vi "WORD report.vi"(7 "Action":T1=enum."Close report", 8 "error in":errorcluster, 10 "Data in":string) -> (0 "error out":errorcluster, 2 "Data out":variant)   [LabVIEW 2015, in "Report.lvlib"]
uses:
  Report.lvlib
  TypeDefs/Report state.ctl
  <vilib>/Utility/NIReport.llb/NI_report.lvclass
  <vilib>/Utility/NIReport.llb/Append Report Text (str wrap).vi
  <vilib>/Utility/NIReport.llb/NI_ReportGenerationCore.lvlib
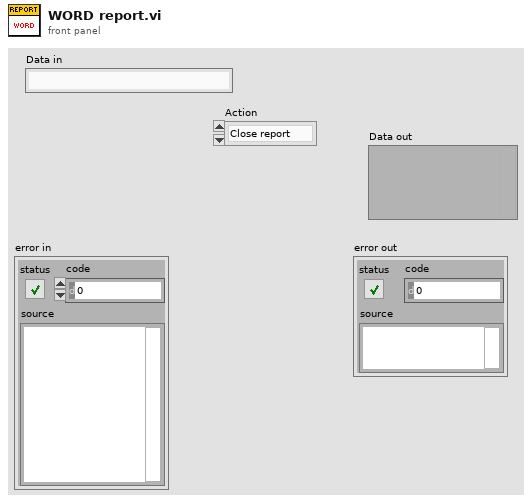
[diagram p1: front panel]
types:
  T1 = typedef "Report.lvlib/Report state.ctl" = enum16{"Create report", "Save data", "Save report", "Available printers", "Print report", "Close report"}
  T2 = enum16{"maximized", "minimized", "normal", "no change"}
  T3 = enum16{"Standard Report", "HTML", "Word", "Excel"}
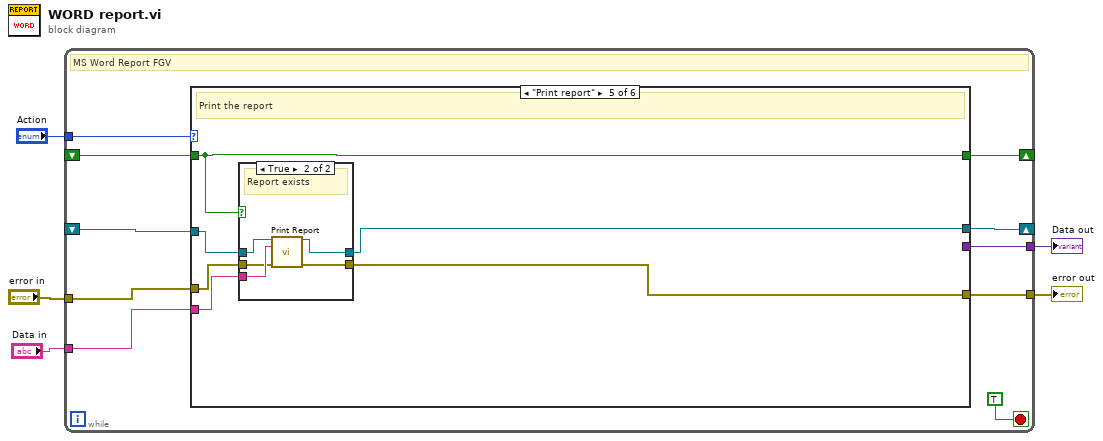
[diagram p0: block diagram]
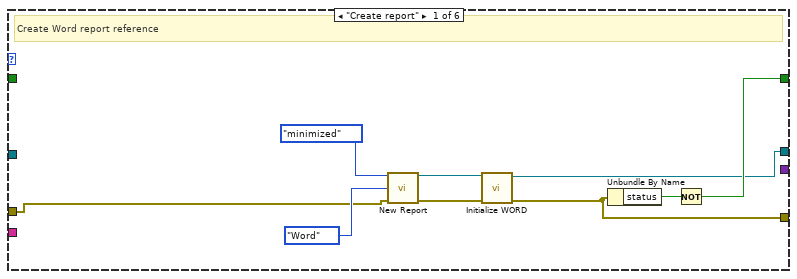
[diagram p2: hidden frame]
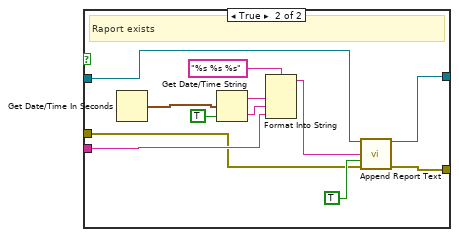
[diagram p4: hidden frame]
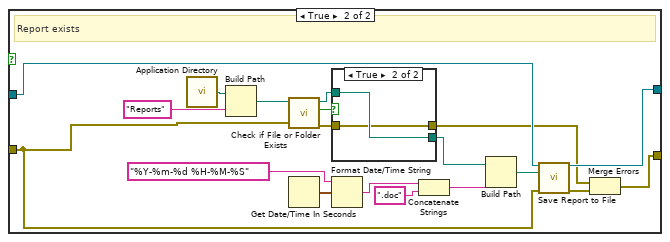
[diagram p6: hidden frame]
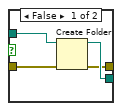
[diagram p7: hidden frame]
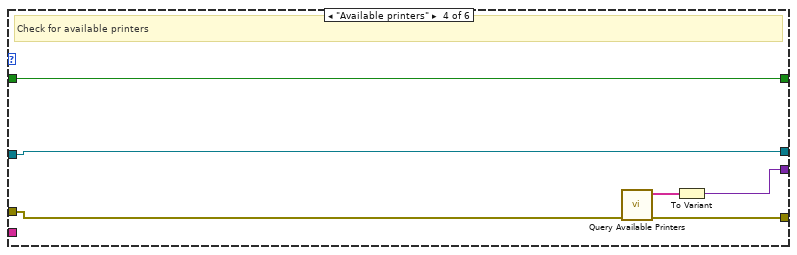
[diagram p8: hidden frame]
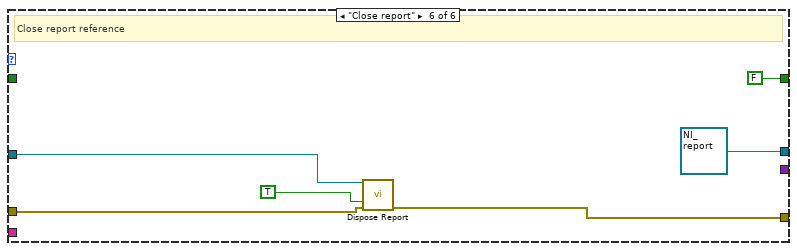
[diagram p10: hidden frame]
diagram:
  n1 = while {
    tunnel: "Action" -> [w13]
    tunnel: "Data in" -> [w14]
    tunnel: "error in" -> [w12]
    tunnel: [w11] -> w3
    tunnel: [w10] -> w1
    shift-right: [w8] -> _
    shift-left: _ -> [w9]
    shift-right: [w7] -> _
    shift-left: _ -> [w6]
    stop <- TRUE stop-if-true
    # "MS Word Report FGV"
    n2 = case shown="\"Print report\"" w13 {
      tunnel: w14 -> [_ w30 _ _ w88 _]
      tunnel: w12 -> [w20 w27 w47 w80 w85 w96]
      tunnel: [_ _ _ w81 _ _] -> w11
      tunnel: [w19 w29 w49 w79 w87 w101] -> w10
      tunnel: w9 -> [_ w28 w48 w78 w86 _]
      tunnel: [w17 w28 w48 w78 w86 FALSE] -> w8
      tunnel: [w16 w25 w45 w77 w83 refnum<class "NI_report.lvclass"> refnum ("report ID")] -> w7
      tunnel: w6 -> [_ w26 w46 w77 w84 w98]
      frame "Create report" {
        # "Create Word report reference"
        n3 = call <vilib>:"New Report.vi"("window state (normal)"=T2."minimized", "report type"=T3."Word", "error in (no error)"=w20) -> ("report out"=w22:refnum<class "NI_report.lvclass">, "error out"=w21:errorcluster)  [unwired: 11 in]
        n4 = call "Initialize WORD.vi"("error in (no error)"=w21, "NI_report in"=w22) -> ("error out"=w19:errorcluster, "NI_report out"=w16:refnum<class "NI_report.lvclass">)  [unwired: 8 in]
        n5 = Unbundle By Name(w19) -> ("status"=w18:bool)
        n6 = Not(x=w18) -> (.not. x?=w17:bool)
      }
      frame "Save data" {
        # "Save date, time and input message (status) in new line"
        n7 = case shown="False" w28 {
          tunnel: w30 -> [_ w37]
          tunnel: [w32 w36] -> w29
          tunnel: w27 -> [w32 w33]
          tunnel: w26 -> [w31 w35]
          tunnel: [w31 w34] -> w25
          frame False {
            # "Report not created"
          }
          frame True {
            # "Raport exists"
            n8 = Get Date/Time In Seconds() -> (seconds since 1Jan1904=w43:timestamp)
            n9 = Get Date/Time String(seconds (now)=w43, want seconds? (F)=TRUE) -> (date string=w41:string, time string=w40:string)  [unwired: 1 in]
            n10 = Format Into String(format string="%s %s %s", w41, w40, w37) -> (resulting string=w38:string)  [unwired: 2 in, 1 out]
            n11 = call-poly <vilib>:"Append Report Text.vi"("report in"=w35, "text"=w38, "append on new line? (F)"=TRUE ("append on new line?"), "error in (no error)"=w33) -> ("report out"=w34:refnum<class "NI_report.lvclass">, "error out"=w36:errorcluster)  [unwired: 8 in, 2 out]
          }
        }
      }
      frame "Save report" {
        # "Save report file on HDD"
        n12 = case shown="False" w48 {
          tunnel: [w51 w52] -> w49
          tunnel: w47 -> [w51 w56]
          tunnel: w46 -> [w50 w58]
          tunnel: [w50 w57] -> w45
          frame False {
            # "Report not created"
          }
          frame True {
            # "Report exists"
            n13 = call <vilib>:"Application Directory.vi"() -> ("Application Directory"=w64:path)
            n14 = Build Path(base path=w64, name or relative path="Reports") -> (appended path=w62:path)
            n15 = call <vilib>:"Check if File or Folder Exists.vi"("error in (no error)"=w56, "path"=w62) -> ("error out"=w55:errorcluster, "file or folder exists?"=w61:bool, "dup path"=w60:path)  [unwired: 7 in]
            n16 = Get Date/Time In Seconds() -> (seconds since 1Jan1904=w69:timestamp)
            n17 = case shown="True" w61 {
              tunnel: w60 -> [w74 w76]
              tunnel: [w73 w76] -> w59
              tunnel: w55 -> [w72 w75]
              tunnel: [w71 w75] -> w54
              frame False {
                n18 = Create Folder(path (use dialog)=w74, error in=w72) -> (created path=w73:path, error out=w71:errorcluster)  [unwired: 1 in, 1 out]
              }
              frame True {
              }
            }
            n19 = Format Date/Time String(time format string (%c)="%Y-%m-%d %H-%M-%S", seconds (now)=w69) -> (date/time string=w67:string)  [unwired: 1 in]
            n20 = Concatenate Strings(w67, ".doc" ("string")) -> (w65:string)
            n21 = Build Path(base path=w59, name or relative path=w65) -> (appended path=w70:path)
            n22 = call-dynamic "Save Report to File.vi"("report in"=w58, "report file path"=w70, "error in (no error)"=w56) -> ("report out"=w57:refnum<class "NI_report.lvclass">, "error out"=w53:errorcluster)  [unwired: 11 in]
            n23 = Merge Errors(w54, w53) -> (w52:errorcluster)
          }
        }
      }
      frame "Available printers" {
        # "Check for available printers"
        n24 = call <vilib>:"Query Available Printers.vi"("error in (no error)"=w80) -> ("error out"=w79:errorcluster, "system configured printers"=w82:string[])  [unwired: 8 in, 1 out]
        n25 = To Variant(anything=w82) -> (Variant=w81:variant)
      }
      frame "Print report" {
        # "Print the report"
        n26 = case shown="True" w86 {
          tunnel: w88 -> [_ w95]
          tunnel: [w90 w94] -> w87
          tunnel: w85 -> [w90 w91]
          tunnel: w84 -> [w89 w93]
          tunnel: [w89 w92] -> w83
          frame False {
            # "Report not created"
          }
          frame True {
            # "Report exists"
            n27 = call-dynamic "Print Report.vi"("report in"=w93, "printer name (default)"=w95, "error in (no error)"=w91) -> ("report out"=w92:refnum<class "NI_report.lvclass">, "error out"=w94:errorcluster)  [unwired: 11 in]
          }
        }
      }
      frame "Close report" {
        # "Close report reference"
        n28 = call-dynamic "Dispose Report.vi"("report in"=w98, "save changes? (F)"=TRUE, "error in (no error)"=w96) -> ("error out"=w101:errorcluster)  [unwired: 12 in]
      }
    }
  }
  "error out" <- w1
  "Data out" <- w3
